vi "_USB_CAN_GLOBAL_.vi"() -> ()   [LabVIEW 2011]
panel:
  out "close":bool
  in  "Disp-HL":bool=TRUE
  in  "R-Enb":bool=TRUE
  out "S-Cnt":i64
  in  "S-Cancel":bool
  out "open":bool
  in  "S-Enable":bool=TRUE
  in  "R-Enable":bool=TRUE
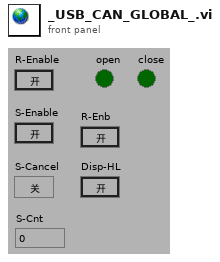
[diagram p1: front panel]
diagram:
